vi "Check for valid serial port.vi"(2 "Serial Port Name":string, 3 "PS Communication Port In":string) -> (0 "Valid Serial Port":bool, 1 "PS Communication Port out":refnum<visa-resource-name>)   [LabVIEW 2019]
uses:
  <vilib>/regexp/Match Regular Expression.xnode
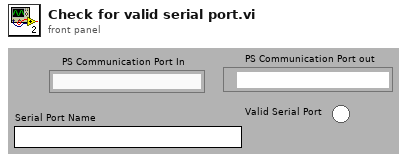
[diagram p1: front panel]
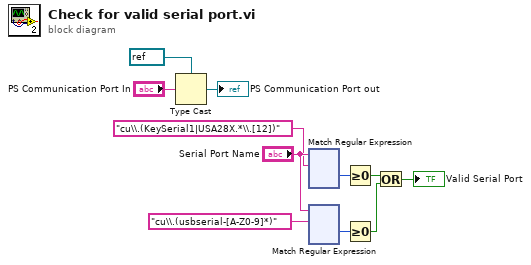
[diagram p0: block diagram]
diagram:
  n1 = Type Cast(type=refnum<visa-resource-name> refnum ("VISA resource name"), x="PS Communication Port In") -> (*(type *) &x=→"PS Communication Port out":refnum<visa-resource-name>)
  n2 = xnode "Match Regular Expression"("input string"="Serial Port Name", "regular expression"="cu\\.(KeySerial1|USA28X.*\\.[12])" ("input string")) -> ("offset past match"=w4:i32)  [unwired: 4 in, 4 out]
  n3 = xnode "Match Regular Expression"("input string"="Serial Port Name", "regular expression"="cu\\.(usbserial-[A-Z0-9]*)" ("input string")) -> ("offset past match"=w3:i32)  [unwired: 4 in, 4 out]
  n4 = Greater Or Equal To 0?(x=w4) -> (x >= 0?=w5:bool)
  n5 = Greater Or Equal To 0?(x=w3) -> (x >= 0?=w1:bool)
  n6 = Or(x=w5, y=w1) -> (x .or. y?=→"Valid Serial Port":bool)
